vi "Giris (SubVI).vi"() -> (0 "Type 2":string, 1 "OKTO":bool, 2 "Username 2":string)   [LabVIEW 2009]
uses:
  <vilib>/Utility/file.llb/Read From Spreadsheet File (string).vi
panel:
  out "Type":string
  in  "Password":string
  in  "Username":string
  in  "OK":bool caption="OK2"
  in  "Cancel":bool
  # "Please enter the username and password"
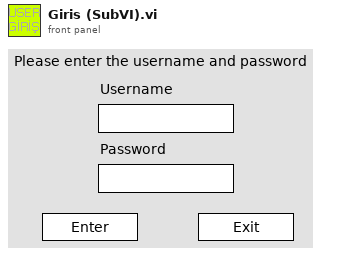
[diagram p1: front panel]
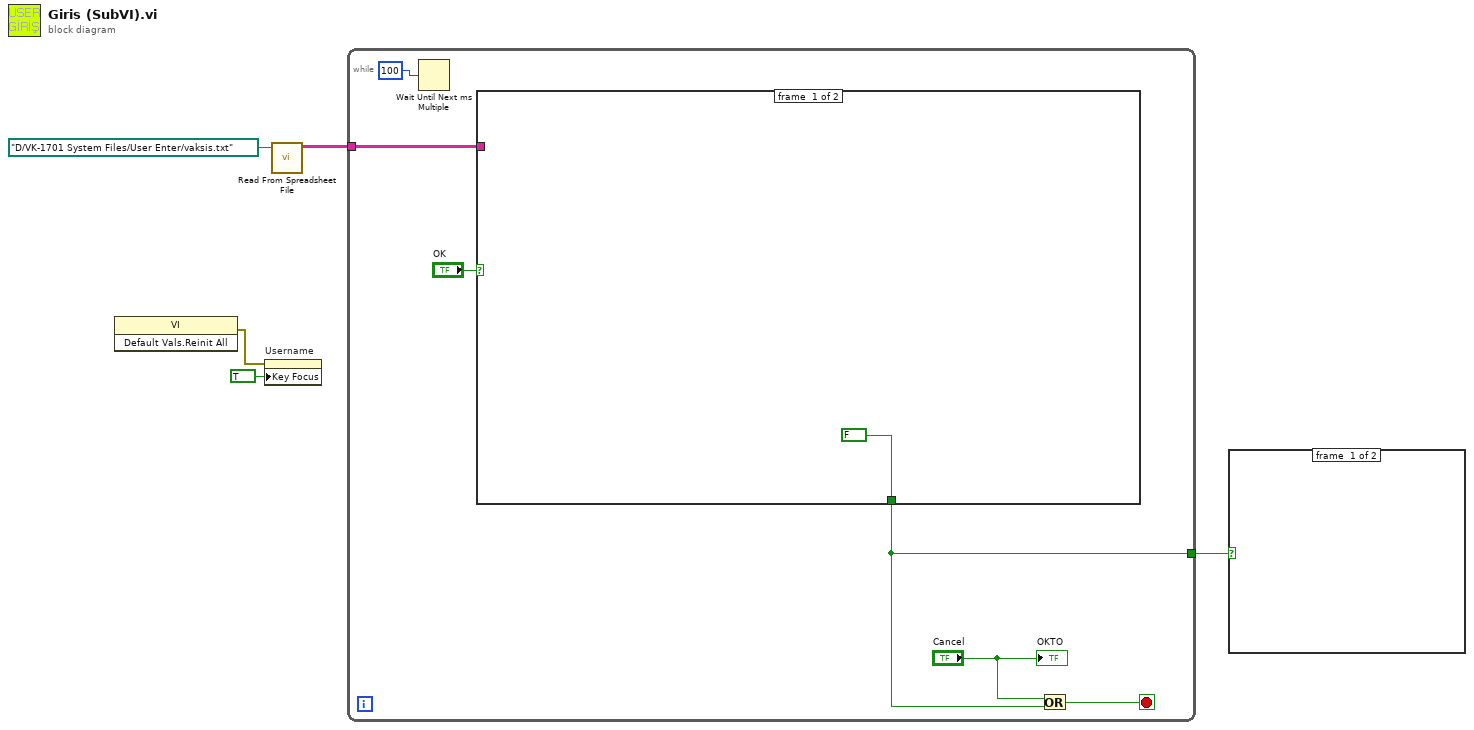
[diagram p0: block diagram]
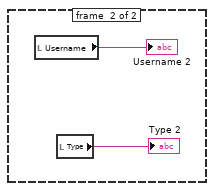
[diagram p2: hidden frame]
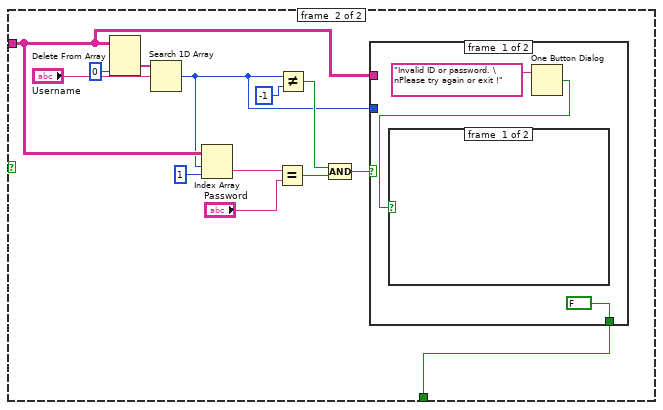
[diagram p3: hidden frame]
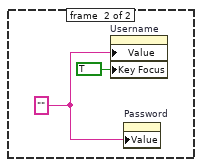
[diagram p4: hidden frame]
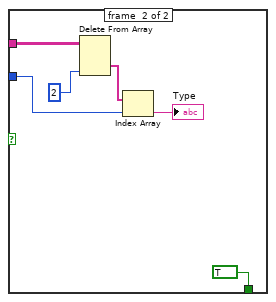
[diagram p5: hidden frame]
diagram:
  n1 = invoke class="VI" method="Default Vals.Reinit All"() -> (error out=w2:errorcluster)  [unwired: 3 in, 2 out]
  n2 = property on="Username" class="Str"(error in=w2, "Key Focus"=TRUE) -> ()  [unwired: 1 in, 2 out]
  n3 = call-poly <vilib>:"Read From Spreadsheet File.vi"("file path (dialog if empty)"=path "D:/VK-1701 System Files/User Enter/vaksis.txt" ("Path")) -> ("all rows"=w4:string[][])  [unwired: 6 in, 4 out]
  n4 = while {
    tunnel: w4 -> [w11]
    tunnel: [w8] -> w3
    stop <- w10 stop-if-true
    n5 = Wait Until Next ms Multiple(millisecond multiple=100) -> ()  [unwired: 1 out]
    n6 = case shown="True" "OK" {
      tunnel: w11 -> [_ w17]
      tunnel: [FALSE w18] -> w8
      frame #0 {
      }
      frame #1 {
        n7 = Delete From Array(array=w17, index (col)=0 ("disabled index (col)")) -> (deleted portion=w23:string[])  [unwired: 2 in, 1 out]
        n8 = Search 1D Array(1D array=w23, element="Username") -> (index of element=w15:i32)  [unwired: 1 in]
        n9 = Index Array(array=w17, index (row)=w15, index (col)=1 ("disabled index (col)")) -> (element=w14:string)
        n10 = Equal?(x=w14, y="Password") -> (x = y?=w20:bool)
        n11 = Not Equal?(x=w15, y=-1) -> (x != y?=w21:bool)
        n12 = Compound Arithmetic op=AND(w21, w20) -> (w19:bool)
        n13 = case shown="True" w19 {
          tunnel: [FALSE TRUE] -> w18
          tunnel: w15 -> [_ w32]
          tunnel: w17 -> [_ w34]
          frame #0 {
            n14 = One Button Dialog(message="Invalid ID or password. \nPlease try again or exit !") -> (true=w26:bool)  [unwired: 1 in]
            n15 = case shown="True" w26 {
              frame #0 {
              }
              frame #1 {
                w30 = "" ("Password")
                n16 = property on="Username" class="Str"("Value"=w30, "Key Focus"=TRUE) -> ()  [unwired: 2 in, 2 out]
                n17 = property on="Password" class="Str"("Value"=w30) -> ()  [unwired: 2 in, 2 out]
              }
            }
          }
          frame #1 {
            n18 = Delete From Array(array=w34, index (col)=2 ("disabled index (col)")) -> (deleted portion=w33:string[])  [unwired: 2 in, 1 out]
            n19 = Index Array(array=w33, index=w32) -> (element=→"Type":string)
          }
        }
      }
    }
    n20 = Or(x="Cancel", y=w8) -> (x .or. y?=w10:bool)
    "OKTO" <- "Cancel"
  }
  n21 = case shown="True" w3 {
    frame #0 {
    }
    frame #1 {
      n22 = local read "Username"() -> (→"Username 2":string)
      n23 = local read "Type"() -> (→"Type 2":string)
    }
  }
